vi "ConvertMeasureToUnitValue.vi"(10 "digit":u8, 11 "value":dbl format="%#_6f") -> (3 "result":string)   [LabVIEW 2018, in "Library-DataConvert.lvlib"]
uses:
  Library-DataConvert.lvlib
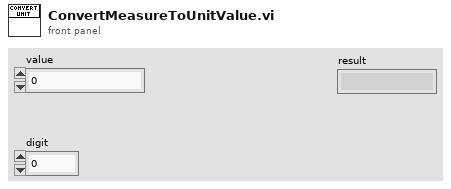
[diagram p1: front panel]
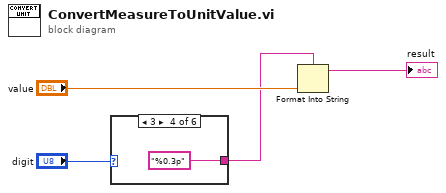
[diagram p0: block diagram]
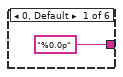
[diagram p2: hidden frame]
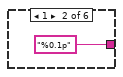
[diagram p3: hidden frame]
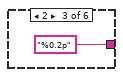
[diagram p4: hidden frame]
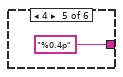
[diagram p5: hidden frame]
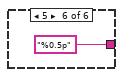
[diagram p6: hidden frame]
diagram:
  n1 = case shown="3" "digit" {
    tunnel: ["%0.0p" ("포맷 문자열") "%0.1p" ("포맷 문자열") "%0.2p" ("포맷 문자열") "%0.3p" ("포맷 문자열") "%0.4p" ("포맷 문자열") "%0.5p" ("포맷 문자열")] -> w1
    frame 0, Default {
    }
    frame 1 {
    }
    frame 2 {
    }
    frame 3 {
    }
    frame 4 {
    }
    frame 5 {
    }
  }
  n2 = Format Into String(format string=w1, "value") -> (resulting string=→"result":string)  [unwired: 2 in, 1 out]
